vi "Create Power Sweep Evals.vi"(8 "error in (no error)":errorcluster, 11 "ModSweep in":refnum<class "Power Sweep.lvclass">) -> (0 "error out":errorcluster, 2 "Evaluations Out":T1[](array[typedef]) {"Low Limit" format="%#_13g"; "SI Scaling" items=["femto"=-15, "pico"=-12, "nano"=-9, "micro"=-6, "milli"=-3, "percent"=-2, ""=0, "kilo"=3, "mega"=6, "giga"=9, "tera"=12]}, 3 "ModSweep out":refnum<class "Power Sweep.lvclass">)   [LabVIEW 2018, in "Power Sweep.lvlib" / "Power Sweep.lvclass"]
uses:
  Power Sweep.lvclass
  C:/Sequence Automation/Plugins/Measurement Interface.lvlibp/Measurement Interface.lvclass
  Plugins/TestStand API Tools (TSAT).lvlibp/Evaluation Actions/Includes/Controls/TSAT Evaluation.ctl
  Plugins/TestStand API Tools (TSAT).lvlibp/Evaluation Actions/Includes/Controls/TSAT Eval SI Unit Scaling.ctl
  Plugins/TestStand API Tools (TSAT).lvlibp/Evaluation Actions/Includes/Controls/TSAT Evaluation Type.ctl
  Power Sweep.lvclass/Power Sweep.ctl
  Plugins/Measurement Interface.lvlibp/Private Methods/Measurement Name/Read Measurement Name.vi
  Read DC Pins.vi
  Plugins/Measurement Interface.lvlibp/Private Methods/Measurement Parameters/Read Measurement Parameters.vi
  Plugins/String Database.lvlibp/String Database.lvclass
  Plugins/SeqAuto Evaluations.lvlibp/Power Sweep/Power Sweep.lvclass
  Plugins/TestStand API Tools (TSAT).lvlibp/Evaluation Actions/TSAT Evaluation Actions.lvlib
  Plugins/Test Number and Bin Generator.lvlibp/Test Number and Bin Generator/Test Number and Bin Generator.lvclass
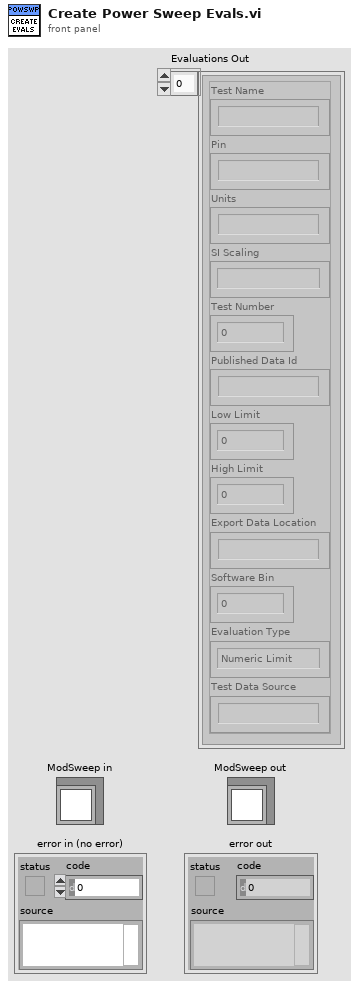
[diagram p1: front panel]
types:
  T1 = typedef "TestStand API Tools (TSAT).lvlibp/TSAT Evaluation Actions.lvlib/TSAT Evaluation.ctl" = cluster{"Test Name":string, "Pin":string, "Units":string, "SI Scaling":T2, "Test Number":i32, "Published Data Id":string, "Low Limit":dbl, "High Limit":dbl, "Export Data Location":string, "Software Bin":i64, "Evaluation Type":T3, "Test Data Source":string}
  T2 = typedef "TestStand API Tools (TSAT).lvlibp/TSAT Evaluation Actions.lvlib/TSAT Eval SI Unit Scaling.ctl" = i16
  T3 = typedef "TestStand API Tools (TSAT).lvlibp/TSAT Evaluation Actions.lvlib/TSAT Evaluation Type.ctl" = enum16{"Numeric Limit", "Pass/Fail", "None"}
  T4 = typedef "Test Number and Bin Generator.lvlibp/Test Number and Bin Generator.lvclass/Session Handle.ctl" = refnum<data-value>
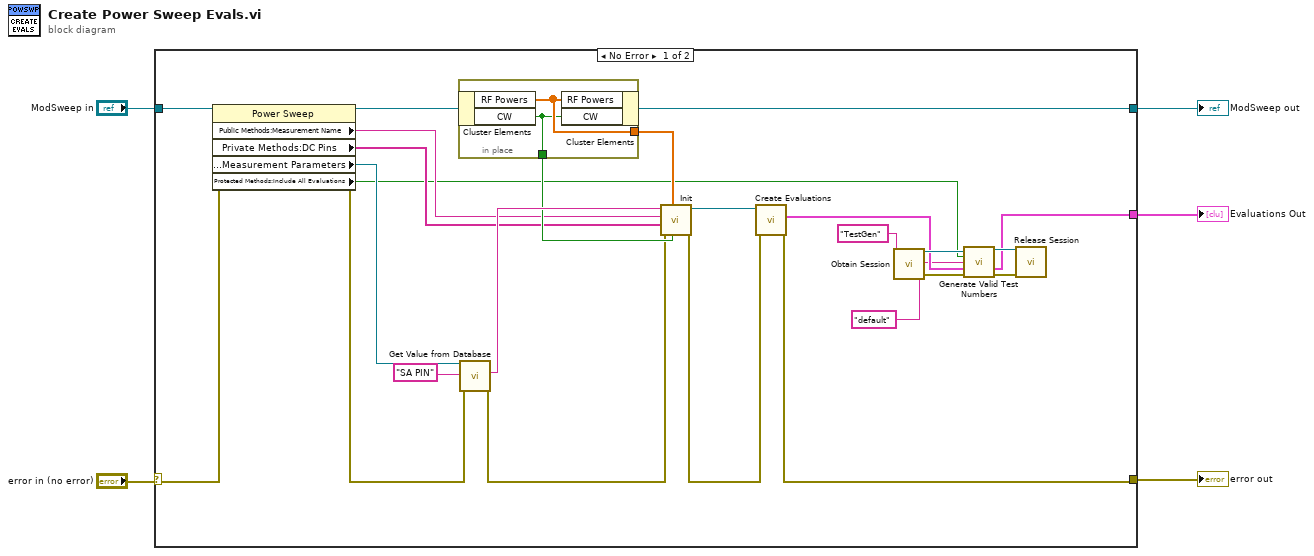
[diagram p0: block diagram]
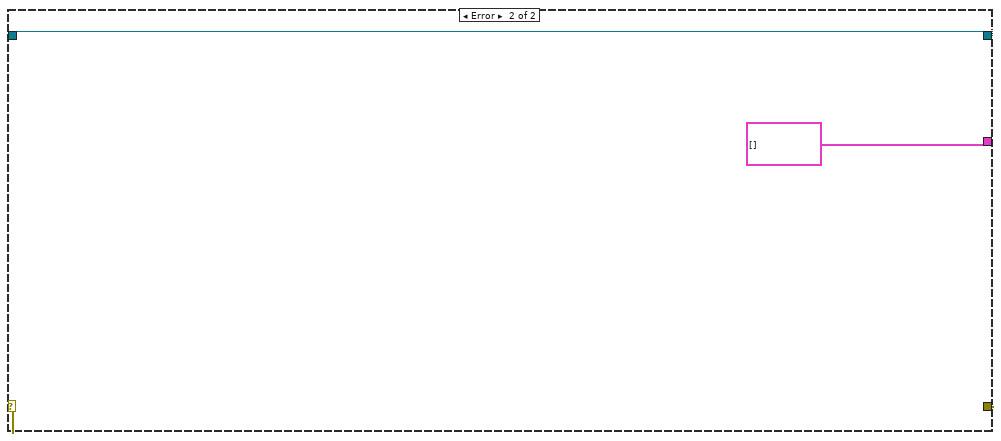
[diagram p2: hidden frame]
diagram:
  n1 = case shown="No Error" "error in (no error)" {
    selector: "error in (no error)" -> [w30 w35]
    tunnel: [w7 w35] -> w4
    tunnel: [w27 w34] -> w2
    tunnel: "ModSweep in" -> [w29 w34]
    tunnel: [w16 T1[] []] -> w1
    frame No Error {
      n2 = property class="Power Sweep"(reference=w29, error in=w30) -> (reference out=w28:refnum<class "Power Sweep.lvclass">, error out=w24:errorcluster, "Public Methods:Measurement Name"=w11:string, "Private Methods:DC Pins"=w10:string[], "Protected Methods:Measurement Parameters"=w25:refnum<class "String Database.lvclass">, "Protected Methods:Include All Evaluations"=w6:bool)
      n3 = in-place {
        in-place-border: [w32] -> w26
        in-place-border: [w31] -> w14
        n4 = in-place-cluster #1(w28) -> ("RF Powers"=w32:dbl[], "CW"=w31:bool)
        n5 = in-place-cluster #1("RF Powers"=w32, "CW"=w31) -> (w27:refnum<class "Power Sweep.lvclass">)
      }
      n6 = call "Get Value from Database.vi"("error in (no error)"=w24, "Entry Name"="SA PIN", "Message in"=w25) -> ("error out"=w9:errorcluster, "Entry Value"=w22:string)  [unwired: 5 in, 2 out]
      n7 = call "Init.vi"("CW?"=w14, "RF Powers"=w26, "error in (no error)"=w9, "DC Pins"=w10, "Measurement Name"=w11, "SA Pin"=w22) -> ("error out"=w8:errorcluster, "ModSweep Gain out"=w12:refnum<class "Power Sweep.lvclass">)  [unwired: 4 in]
      n8 = call-dynamic "Create Evaluations.vi"("error in (no error)"=w8, "Power Sweep Eval In"=w12) -> ("error out"=w7:errorcluster, "Evaluations Out"=w15:T1[])  [unwired: 7 in, 1 out]
      n9 = call "Obtain Session.vi"("Session  Name ()"="TestGen") -> ("Session Handle"=w18:T4, "error out"=w19:errorcluster)  [unwired: 13 in]
      n10 = call "Generate Valid Test Numbers.vi"("Session Handle in"=w18, "Include All Evaluations?"=w6, "Test Group"="default", "Evaluations In"=w15, "error in (no error)"=w19) -> ("Session Handle out"=w20:T4, "Evaluations Out"=w16:T1[], "error out"=w21:errorcluster)  [unwired: 8 in]
      n11 = call "Release Session.vi"("Session Handle"=w20, "error in (no error)"=w21) -> ()  [unwired: 13 in, 1 out]
    }
    frame Error {
    }
  }
  "error out" <- w4
  "ModSweep out" <- w2
  "Evaluations Out" <- w1
